vi "APIEscribir datos en Google Sheets_boleto.vi"(0 "Cluster":cluster{"hora_entrada":string, "id":string}) -> ()   [LabVIEW 2025]
uses:
  <vilib>/httpClient/POSTBuffer.vi
  <vilib>/httpClient/LabVIEWHTTPClient.lvlib
panel:
  out "write_response":string
  out "write_url":string
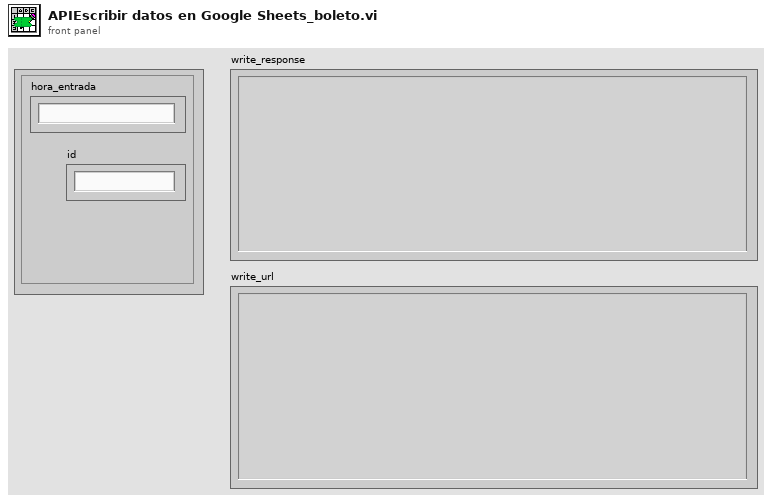
[diagram p1: front panel]
types:
  T1 = typedef "LabVIEWHTTPClient.lvlib/ClientHandle.ctl" = refnum<k1>
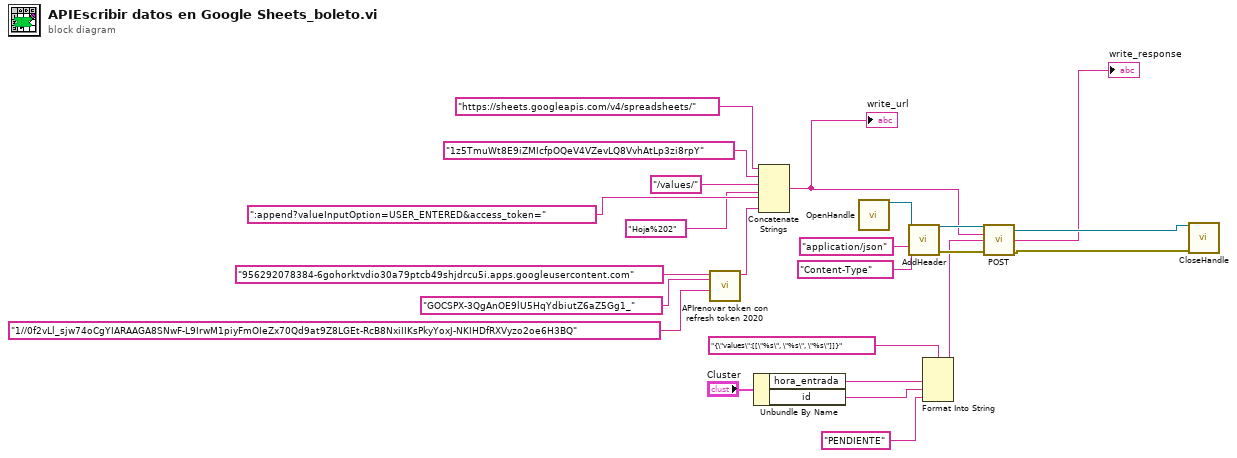
[diagram p0: block diagram]
diagram:
  n1 = call "APIrenovar token con refresh token 2020.vi"("refresh_token"="1//0f2vLl_sjw74oCgYIARAAGA8SNwF-L9IrwM1piyFmOIeZx70Qd9at9Z8LGEt-RcB8NxiIIKsPkyYoxJ-NKIHDfRXVyzo2oe6H3BQ", "client_secret"="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", "client_id"="956292078384-6gohorktvdio30a79ptcb49shjdrcu5i.apps.googleusercontent.com") -> ("access_token"=w7:string)  [unwired: 8 in]
  n2 = Unbundle By Name("Cluster") -> ("hora_entrada"=w3:string, "id"=w2:string)
  n3 = Concatenate Strings("https://sheets.googleapis.com/v4/spreadsheets/", "1z5TmuWt8E9iZMIcfpOQeV4VZevLQ8VvhAtLp3zi8rpY" ("spreadsheet_id"), "/values/", "Hoja%202" ("write_range"), ":append?valueInputOption=USER_ENTERED&access_token=", w7) -> (w12:string)
  "write_url" <- w12
  n4 = call <vilib>:"OpenHandle.vi"() -> ("client handle out"=w19:T1)  [unwired: 14 in, 1 out]
  n5 = call <vilib>:"AddHeader.vi"("client handle"=w19, "header"="Content-Type", "value"="application/json") -> ("client handle out"=w16:T1, "error out"=w15:errorcluster)  [unwired: 11 in]
  n6 = Format Into String(format string="{\"values\":[[\"%s\", \"%s\", \"%s\"]]}", w3, w2, "PENDIENTE" ("input 6")) -> (resulting string=w5:string)  [unwired: 2 in, 1 out]
  n7 = call-poly <vilib>:"POST.vi"("client handle"=w16, "url"=w12, "buffer"=w5, "error in (no error)"=w15) -> ("client handle out"=w14:T1, "body"=→"write_response":string, "error out"=w13:errorcluster)  [unwired: 8 in, 1 out]
  n8 = call <vilib>:"CloseHandle.vi"("client handle"=w14, "error in (no error)"=w13) -> ()  [unwired: 13 in, 1 out]
